vi "Analog read waveform op.vi"() -> ()   [LabVIEW 2014]
uses:
  Control 1.ctl
  <vilib>/LabVIEW Interface for Arduino/LabVIEW Interface for Arduino.lvlib
panel:
  out "Numeric":dbl
  out "Waveform Chart":T1
  in  "?":bool
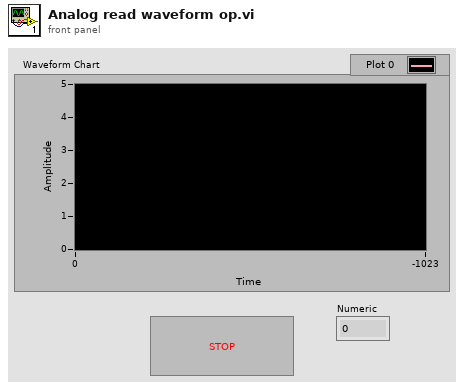
[diagram p1: front panel]
types:
  T1 = typedef "Control 1.ctl" = dbl
  T2 = typedef "LabVIEW Interface for Arduino.lvlib/Arduino Resource.ctl" = cluster{"VISA resource":refnum<visa-resource-name>, "Board Type":T3, "Connection Type":enum8{"USB / Serial"}, "Bytes Per Packet (15)":u8}
  T3 = typedef "LabVIEW Interface for Arduino.lvlib/Board Type.ctl" = enum16{"Uno", "Dimuelanove w/Atmega 328", "Mega 2560"}
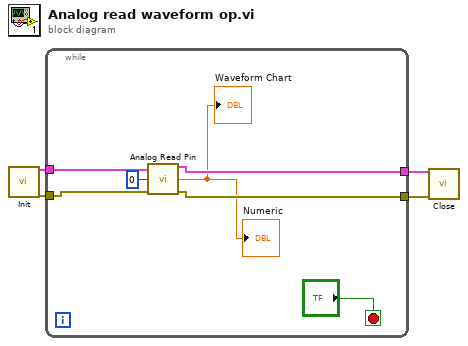
[diagram p0: block diagram]
diagram:
  n1 = call <vilib>:"Init.vi"() -> ("Arduino Resource"=w4:T2, "error out"=w3:errorcluster)  [unwired: 18 in]
  n2 = while {
    tunnel: w4 -> [w10]
    tunnel: w3 -> [w9]
    tunnel: [w8] -> w2
    tunnel: [w7] -> w1
    stop <- "?" stop-if-true
    n3 = call <vilib>:"Analog Read Pin.vi"("Arduino Resource"=w10, "Analog Input Pin (0)"=u8 0, "error in"=w9) -> ("Arduino Resource"=w8:T2, "Voltage"=→"Waveform Chart" →"Numeric":dbl, "error out"=w7:errorcluster)  [unwired: 10 in]
  }
  n4 = call <vilib>:"Close.vi"("Arduino Resource"=w2, "error in"=w1) -> ()  [unwired: 13 in, 1 out]
